vi "PrepForMultiply.vi"(0 "A":T1) -> (1 "Starting Condition":cluster{"digit":i32, i32, i32}, 2 "Working Digits":i32, 3 "Trailing Zeroes":i32, 4 "New Decimal Index":i32)   [LabVIEW 2025]
uses:
  Number.ctl
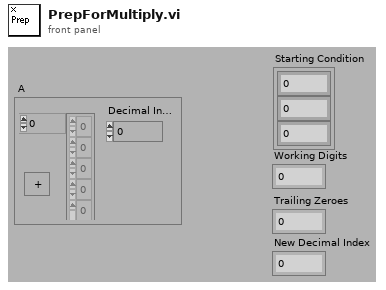
[diagram p1: front panel]
types:
  T1 = typedef "Number.ctl" = cluster{"Array Num":i8[], "Decimal Index":i32, "stop":bool}
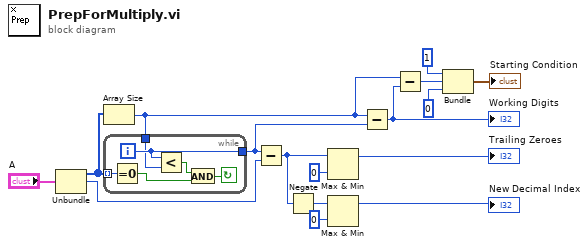
[diagram p0: block diagram]
diagram:
  n1 = Unbundle("A") -> ("Array Num"=w10:i8[], "Decimal Index"=w15:i32)  [unwired: 1 out]
  n2 = Array Size(array=w10) -> (size(s)=w4:i32)
  n3 = while {
    tunnel: w10 -> [w22] mode=indexing
    tunnel: [w18] -> w5
    tunnel: w4 -> [w17]
    i -> [w18]
    stop <- w19 continue-if-true
    n4 = Equal To 0?(x=w22) -> (x = 0?=w21:bool)
    n5 = Less?(x=w18, y=w17) -> (x < y?=w20:bool)
    n6 = And(x=w20, y=w21) -> (x .and. y?=w19:bool)
  }
  n7 = Subtract(x=w5, y=w15) -> (x-y=w6:i32)
  n8 = Negate(x=w6) -> (-x=w12:i32)
  n9 = Max & Min(x=w6, y=0 ("digit")) -> (max(x,y)=→"Trailing Zeroes":i32)  [unwired: 1 out]
  n10 = Max & Min(x=w12, y=0 ("digit")) -> (max(x,y)=→"New Decimal Index":i32)  [unwired: 1 out]
  n11 = Subtract(x=w4, y=w5) -> (x-y=w2:i32)
  "Working Digits" <- w2
  n12 = Subtract(x=w4, y=w2) -> (x-y=w3:i32)
  n13 = Bundle("digit"=1, w3, "digit"=0) -> (→"Starting Condition":cluster{"digit":i32, i32, "digit":i32})  [unwired: 1 in]
